vi "IMULoop.vi"(6 "I2CDevRef 2":T10={"DevStatus"={"status"=FALSE, "code"=0, "source"=""}, "Controller"=enum."Controller 1", "Device Address"=0, "Handle"=0, "I2C Bus"=enum."Invalid"} {"Device Address" format="%.0x"}, 8 "AccelerometerDevRef":T1={"DevStatus"={"status"=FALSE, "code"=0, "source"=""}, "Controller"=enum."Controller 1", "Scaling"={"Gain (VoltsPerG)"=0.0, "Center Voltage"=0.0}, "Analog Channels"={"X-Axis"=enum."Invalid", "Y-Axis"=enum."Invalid", "Z-Axis"=enum."Invalid"}, "I2C Bus"=enum."Invalid", "SPI Bus"=enum."Invalid", "Accel Range"=0, "ADXL345 Axes"={"X-Axis"=FALSE, "Y-Axis"=FALSE, "Z-Axis"=FALSE}, "Handle"=0, "Device Address"=0, "Accel Type"=enum."Analog"} {"Device Address" format="%.0x"; "Accel Range" items=["+/- 2 g", "+/- 4 g", "+/- 8 g", "+/- 16 g"]}) -> ()   [LabVIEW 2014]
uses:
  <vilib>/Rock Robotics/WPI/I2C/WPI_I2CDevRef.ctl
  <vilib>/Rock Robotics/SystemInterfaces/Typedef/FPGA_TypedefDigitalModule.ctl
  <vilib>/Rock Robotics/SystemInterfaces/i2clib/i2c_bus.ctl
  <vilib>/Rock Robotics/WPI/Accelerometer/WPI_AccelerometerDevRef.ctl
  <vilib>/Rock Robotics/SystemInterfaces/Typedef/FPGA_TypedefAnalogModule.ctl
  <vilib>/Rock Robotics/WPI/Accelerometer/WPI_AccelerometerScaling.ctl
  <vilib>/Rock Robotics/WPI/Accelerometer/WPI_AccelerometerAnalogChannels.ctl
  <vilib>/Rock Robotics/SystemInterfaces/AI/FPGA_AIChannel.ctl
  <vilib>/Rock Robotics/SystemInterfaces/spilib/spi_bus.ctl
  <vilib>/Rock Robotics/WPI/Accelerometer/ADXL345 Range.ctl
  <vilib>/Rock Robotics/WPI/Accelerometer/WPI_AccelerometerADXL345 Axes.ctl
  <vilib>/Platform/TimedLoop/XDataNode/timing_clust.ctl
  <vilib>/Platform/TimedLoop/XDataNode/nitl_modes.ctl
  <vilib>/Platform/TimedLoop/XDataNode/wakeup.ctl
  Common Code/IMU Data.ctl
  Common Code/Utilities/Radians to Degrees.vi
  Robot Global Data.vi
  <vilib>/Platform/TimedLoop/XDataNode/XDataNode.xnode
  <vilib>/Platform/TimedLoop/XDataNode/XDNodeRunTimeDep.lvlib
panel:
  # "ADXL345"
  # "Analog"
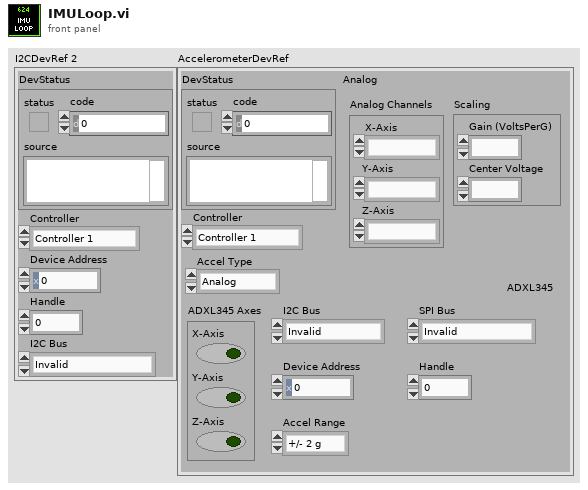
[diagram p1: front panel]
types:
  T1 = typedef "WPI_AccelerometerDevRef.ctl" = cluster{"DevStatus":errorcluster, "Controller":T2, "Scaling":T3, "Analog Channels":T4, "I2C Bus":T6, "SPI Bus":T7, "Accel Range":T8, "ADXL345 Axes":T9, "Handle":i32, "Device Address":u8, "Accel Type":enum16{"Analog", "ADXL345 I2C", "ADXL345 SPI", "Internal"}}
  T2 = typedef "FPGA_TypedefAnalogModule.ctl" = enum16{"Controller 1"}
  T3 = typedef "WPI_AccelerometerScaling.ctl" = cluster{"Gain (VoltsPerG)":dbl, "Center Voltage":dbl}
  T4 = typedef "WPI_AccelerometerAnalogChannels.ctl" = cluster{"X-Axis":T5, "Y-Axis":T5, "Z-Axis":T5}
  T5 = typedef "FPGA_AIChannel.ctl" = enum8{"AI 0", "AI 1", "AI 2", "AI 3", "AI MXP 0", "AI MXP 1", "AI MXP 2", "AI MXP 3", "Invalid"}
  T6 = typedef "i2c_bus.ctl" = enum16{"I2C On-Board", "I2C MXP", "Invalid"}
  T7 = typedef "spi_bus.ctl" = enum16{"SPI On-Board, CS0", "SPI On-Board, CS1", "SPI On-Board, CS2", "SPI On-Board, CS3", "SPI MXP", "Invalid"}
  T8 = typedef "ADXL345 Range.ctl" = u8
  T9 = typedef "WPI_AccelerometerADXL345 Axes.ctl" = cluster{"X-Axis":bool, "Y-Axis":bool, "Z-Axis":bool}
  T10 = typedef "WPI_I2CDevRef.ctl" = cluster{"DevStatus":errorcluster, "Controller":T11, "Device Address":u8, "Handle":i32, "I2C Bus":T6}
  T11 = typedef "FPGA_TypedefDigitalModule.ctl" = enum16{"Controller 1"}
  T12 = typedef "XDNodeRunTimeDep.lvlib/timing_clust.ctl" = cluster{"Expected End [f-1]":u64, "Actual End [f-1]":u64, "Finished Late? [f-1]":bool, "Expected End [i-1]":u64, "Actual End [i-1]":u64, "Finished Late? [i-1]":bool, "Expected Start [i]":u64, "Actual Start [i]":u64, "Expected Start [f]":u64, "Actual Start [f]":u64, "Source Name":string, "Structure Name":string, "Period":i64, "Deadline":i64, "Offset":i64, "Start":i64, "Priority":i32, "Timeout":i32, "Mode":T13, "Wakeup Reason":T14, "Error":errorcluster, "Source Type":string, "Secondary Source Type":string, "Global End Time":u64, "Global Start Time":u64, "Frame Duration":u64, "Iteration Duration":u64, "Assigned CPU":i32, "I/O Scan Engine Mode":u32}
  T13 = typedef "XDNodeRunTimeDep.lvlib/nitl_modes.ctl" = enum32{"No Change", "Process missed periods, maintain original phase", "Discard missed periods, maintain original phase", "Process missed periods, ignore original phase", "Discard missed periods, ignore original phase"}
  T14 = typedef "XDNodeRunTimeDep.lvlib/wakeup.ctl" = enum32{"Normal", "Aborted", "Asynchronous wakeup", "Timing source error", "Timed loop error", "Timeout"}
  T15 = typedef "IMU Data.ctl" = cluster{"Pitch":sgl, "Roll":sgl, "Yaw":sgl}
  T16 = cluster{"X-Axis":dbl, "Y-Axis":dbl, "Z-Axis":dbl}
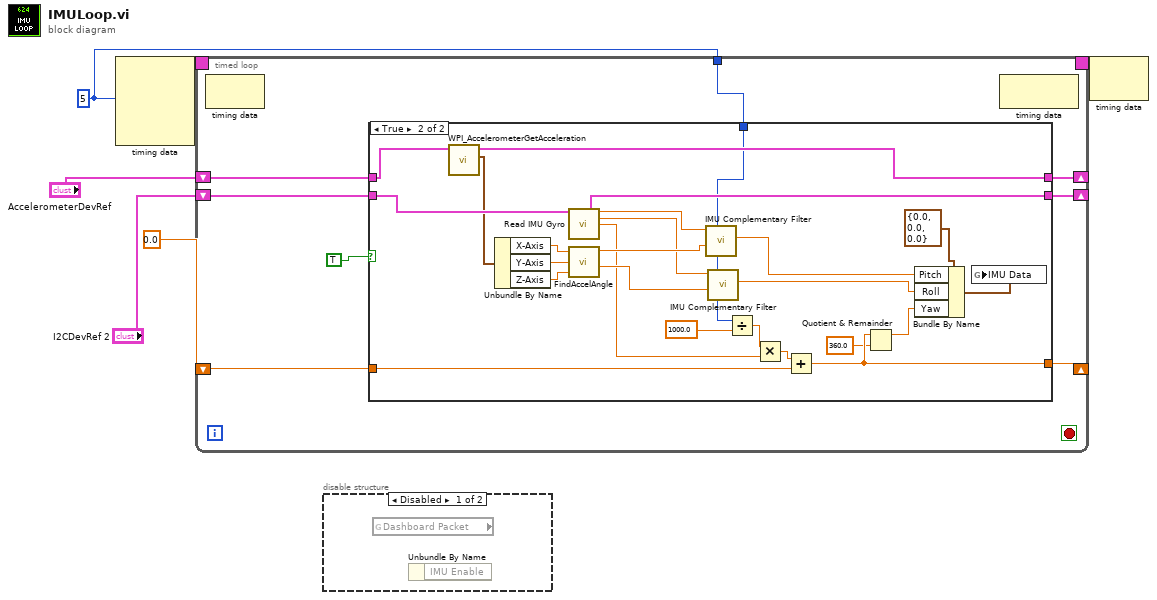
[diagram p0: block diagram]
diagram:
  w2 = u16 5 ("Period")
  n1 = node-c288(w2) -> (w6:T12)  [unwired: 3 in]
  n2 = timed-loop {
    timing: w6 -> [_]
    timing-out: [_] -> w5
    shift-right: [w14] -> _
    shift-left: "I2CDevRef 2" -> [w13]
    shift-right: [w11] -> _
    shift-left: "AccelerometerDevRef" -> [w12]
    tunnel: w2 -> [w9]
    shift-right: [w8] -> _
    shift-left: 0.0 -> [w10]
    stop <- _ stop-if-true
    n3 = node-c288() -> ()  [unwired: 1 in, 1 out]
    n4 = case shown="True" TRUE {
      tunnel: [w16 w39] -> w14
      tunnel: w13 -> [w16 w38]
      tunnel: w12 -> [w17 w36]
      tunnel: [w17 w35] -> w11
      tunnel: w10 -> [w15 w34]
      tunnel: w9 -> [_ w29]
      tunnel: [w15 w20] -> w8
      frame False {
      }
      frame True {
        n5 = call <vilib>:"WPI_AccelerometerGetAcceleration.vi"("AccelerometerDevRef"=w36) -> ("Accelerations"=w37:T16, "AccelerometerDevRef"=w35:T1)  [unwired: 8 in, 1 out]
        n6 = Unbundle By Name(w37) -> ("X-Axis"=w40:dbl, "Y-Axis"=w41:dbl, "Z-Axis"=w42:dbl)
        n7 = call "Read IMU Gyro.vi"("I2CDevRef"=w38) -> ("I2CDevRef 2"=w39:T10, "X"=w33:dbl, "Y"=w31:dbl, "Z"=w26:dbl)  [unwired: 8 in, 3 out]
        n8 = call "FindAccelAngle.vi"("Z"=w42, "Y"=w41, "X"=w40) -> ("Roll"=w30:dbl, "Pitch"=w32:dbl)  [unwired: 4 in]
        n9 = call "IMU Complementary Filter.vi"("dt (ms)"=w29, "Accelerometer Angle"=w32, "Angular vel (gyro, deg/sec)"=w33) -> ("Current Angle"=w21:dbl)  [unwired: 8 in]
        n10 = call "IMU Complementary Filter.vi"("dt (ms)"=w29, "Accelerometer Angle"=w30, "Angular vel (gyro, deg/sec)"=w31) -> ("Current Angle"=w22:dbl)  [unwired: 8 in]
        n11 = Divide(x=w29, y=1000.0) -> (x/y=w27:dbl)
        n12 = Multiply(x=w27, y=w26) -> (x*y=w25:dbl)
        n13 = Add(x=w25, y=w34) -> (x+y=w20:dbl)
        n14 = Quotient & Remainder(x=w20, y=360.0) -> (x-y*floor(x/y)=w18:dbl)  [unwired: 1 out]
        n15 = Bundle By Name(cluster=T15 {"Pitch"=0.0, "Roll"=0.0, "Yaw"=0.0} ("IMU Data"), "Pitch"=w21, "Roll"=w22, "Yaw"=w18) -> (w23:T15)
        n16 = global write "Robot Global Data.vi" "IMU Data"(w23) -> ()
      }
    }
    n17 = node-c288() -> ()  [unwired: 1 in, 1 out]
  }
  n18 = disable-structure shown="Disabled" {
    frame Disabled {
      n19 = global read "Robot Global Data.vi" "Dashboard Packet"() -> ()  [unwired: 1 out]
      n20 = Unbundle By Name() -> ()  [unwired: 1 in, 1 out]
    }
    frame Enabled {
    }
  }
  n21 = node-c288(w5) -> ()  [unwired: 1 out]
